vi "Initiate Measurement.vi"(0 "RS232 Port In":refnum<visa-resource-name>="COM1", 1 "Sensor Address In":string="0", 2 "Measurement Type In (Normal)":i32(ring) items=["Normal", "Concurrent", "Continuous"], 5 "Error In (No Error)":errorcluster, 6 "CRC In (False)":bool, 8 "Parameter In (0)":i32(ring) items=["0", "1", "2", "3", "4", "5", "6", "7", "8", "9"]) -> (10 "Parameter Out":i32(ring) items=["0", "1", "2", "3", "4", "5", "6", "7", "8", "9"], 12 "CRC Out":bool, 14 "RS232 Port Out":refnum<visa-resource-name>="COM1", 15 "Sensor Address Out":string="a", 16 "Measurement Type Out":i32(ring) items=["Normal", "Concurrent", "Continuous"], 17 "Number of Measurements":i32, 18 "Max Acquisition Time (sec)":i32, 19 "Error Out":errorcluster)   [LabVIEW 2016, in "SDI-12.lvlib"]
doc: "Creates and sends the Start Measurement command to the sensor. Scans the sensor's reply for the maximum amount of time for the measurement to complete, and the number of measurements that it will return.\n\nThis VI should only be called for Normal and Concurrent Measurements. Do not call with Continuous Measurements."
uses:
  SDI-12.lvlib
panel:
  out "loop":i32
  out "read buffer":string
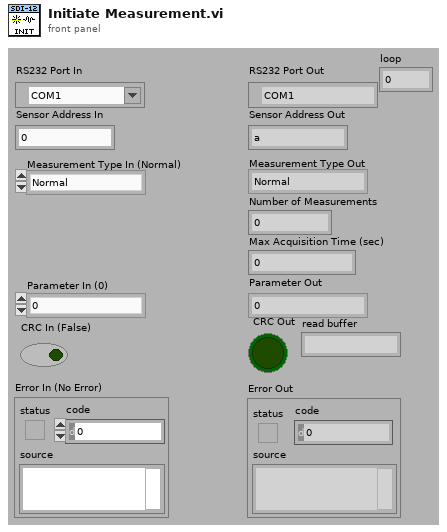
[diagram p1: front panel]
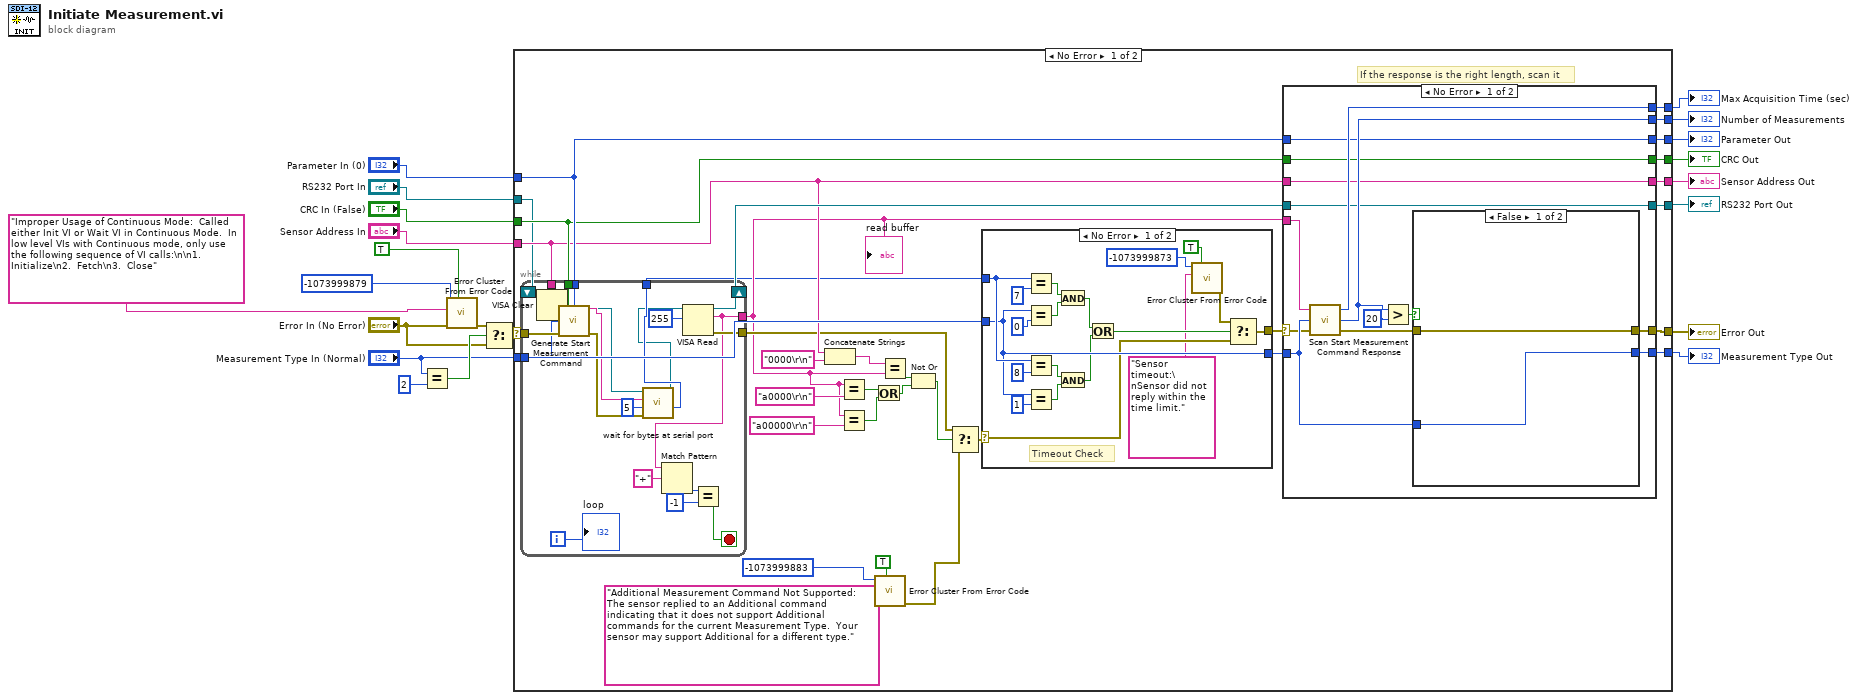
[diagram p0: block diagram]
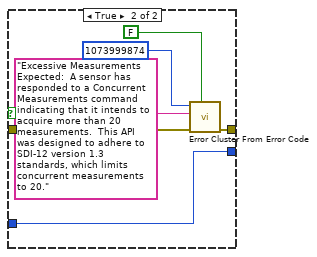
[diagram p3: hidden frame]
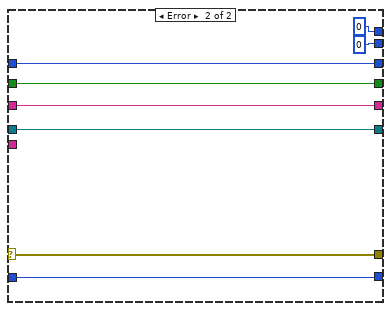
[diagram p4: hidden frame]
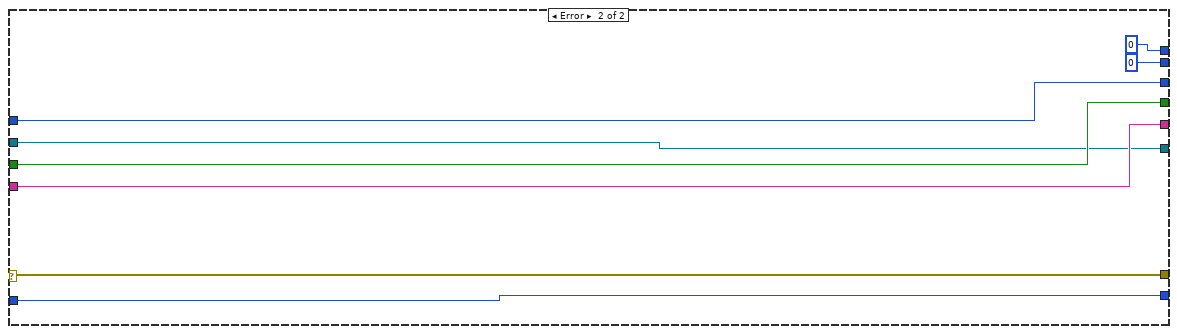
[diagram p5: hidden frame]
diagram:
  n1 = Equal?(x="Measurement Type In (Normal)", y=2) -> (x = y?=w16:bool)
  n2 = call <vilib>:"Error Cluster From Error Code.vi"("show call chain? (False)"=TRUE ("Error?"), "error in (no error)"="Error In (No Error)", "error message (\"\")"="Improper Usage of Continuous Mode:  Called either Init VI or Wait VI in Continuous Mode.  In low level VIs with Continuous mode, only use the following sequence of VI calls:\n\n1.  Initialize\n2.  Fetch\n3.  Close" ("error message (\"\")"), "error code (0)"=-1073999879 ("error code")) -> ("error out"=w15:errorcluster)  [unwired: 5 in]
  n3 = Select(t=w15, s=w16, f="Error In (No Error)") -> (s? t:f=w14:errorcluster)
  n4 = case shown="No Error" w14 {
    selector: w14 -> [w55 w135]
    tunnel: [w54 w135] -> w21
    tunnel: "Measurement Type In (Normal)" -> [w34 w134]
    tunnel: "RS232 Port In" -> [w22 w128]
    tunnel: "Parameter In (0)" -> [w50 w131]
    tunnel: "CRC In (False)" -> [w48 w130]
    tunnel: "Sensor Address In" -> [w31 w129]
    tunnel: [w53 w134] -> w7
    tunnel: [w52 0 ("Number of Measurements")] -> w6
    tunnel: [w51 0 ("Max Acquisition Time")] -> w5
    tunnel: [w49 w131] -> w4
    tunnel: [w47 w130] -> w3
    tunnel: [w46 w129] -> w2
    tunnel: [w44 w128] -> w1
    frame No Error {
      # "If the response is the right length, scan it"
      n5 = while {
        tunnel: w55 -> [w76]
        tunnel: w50 -> [w74]
        tunnel: w48 -> [w73]
        tunnel: w34 -> [w71]
        tunnel: w31 -> [w70]
        tunnel: [w69] -> w29
        tunnel: [w62] -> w28
        tunnel: [w68] -> w23
        shift-right: [w72] -> w45
        shift-left: w22 -> [w66]
        i -> [w57]
        stop <- w58 stop-if-true
        n6 = VISA Clear(VISA resource name=w66) -> (VISA resource name out=w56:refnum<visa-resource-name>)  [unwired: 1 in, 1 out]
        n7 = call "Generate Start Measurement Command.vi"("Sensor Address In"=w70, "CRC (False)"=w73, "Parameter (0)"=w74, "Measurement Type In (Normal)"=w71, "Error In (No Error)"=w76) -> ("Command"=w64:string, "Error Out"=w65:errorcluster)  [unwired: 9 in]
        n8 = call "wait for bytes at serial port.vi"("error in (no error)"=w65, "lower limit"=5, "String"=w64, "VISA Refnum in"=w56) -> ("return count"=w68:u32, "VISA Refnum out"=w67:refnum<visa-resource-name>)  [unwired: 4 in, 2 out]
        n9 = VISA Read(VISA resource name=w67, byte count=u32 255) -> (VISA resource name out=w72:refnum<visa-resource-name>, read buffer=w62:string, error out=w69:errorcluster)  [unwired: 1 in, 1 out]
        n10 = Match Pattern(string=w62, regular expression="+") -> (offset past match=w60:i32)  [unwired: 1 in, 3 out]
        n11 = Equal?(x=w60, y=-1) -> (x = y?=w58:bool)
        "loop" <- w57
      }
      "read buffer" <- w28
      n12 = Concatenate Strings(w31, "0000\r\n") -> (w38:string)
      n13 = Equal?(x=w28, y="a0000\r\n" ("read buffer")) -> (x = y?=w26:bool)
      n14 = Equal?(x=w28, y="a00000\r\n" ("read buffer")) -> (x = y?=w25:bool)
      n15 = Or(x=w26, y=w25) -> (x .or. y?=w24:bool)
      n16 = call <vilib>:"Error Cluster From Error Code.vi"("show call chain? (False)"=TRUE, "error message (\"\")"="Additional Measurement Command Not Supported:  The sensor replied to an Additional command indicating that it does not support Additional commands for the current Measurement Type.  Your sensor may support Additional for a different type." ("error message (\"\")"), "error code (0)"=-1073999883 ("error code")) -> ("error out"=w30:errorcluster)  [unwired: 6 in]
      n17 = Equal?(x=w38, y=w28) -> (x = y?=w37:bool)
      n18 = Not Or(1:w24, 2:w37) -> (0:w36:bool)
      n19 = Select(t=w29, s=w36, f=w30) -> (s? t:f=w35:errorcluster)
      n20 = case shown="No Error" w35 {
        selector: w35 -> [w83 w96]
        tunnel: w23 -> [w89 _]
        tunnel: w34 -> [w87 w97]
        tunnel: [w87 w97] -> w33
        tunnel: [w77 w96] -> w32
        frame No Error {
          # "Timeout Check"
          n21 = Equal?(x=w89, y=u32 7) -> (x = y?=w94:bool)
          n22 = Equal?(x=w87, y=0) -> (x = y?=w92:bool)
          n23 = Equal?(x=w89, y=u32 8) -> (x = y?=w91:bool)
          n24 = Equal?(x=w87, y=1) -> (x = y?=w90:bool)
          n25 = And(x=w94, y=w92) -> (x .and. y?=w85:bool)
          n26 = And(x=w91, y=w90) -> (x .and. y?=w84:bool)
          n27 = Or(x=w85, y=w84) -> (x .or. y?=w82:bool)
          n28 = call <vilib>:"Error Cluster From Error Code.vi"("show call chain? (False)"=TRUE ("Error?"), "error message (\"\")"="Sensor timeout:\nSensor did not reply within the time limit." ("error message (\"\")"), "error code (0)"=-1073999873 ("error code")) -> ("error out"=w78:errorcluster)  [unwired: 6 in]
          n29 = Select(t=w78, s=w82, f=w83) -> (s? t:f=w77:errorcluster)
        }
        frame Error {
        }
      }
      n30 = case shown="No Error" w32 {
        selector: w32 -> [w98 w120]
        tunnel: w28 -> [w109 _]
        tunnel: w33 -> [w106 w121]
        tunnel: [w107 w120] -> w54
        tunnel: [w105 w121] -> w53
        tunnel: [w104 0 ("Number of Measurements")] -> w52
        tunnel: [w103 0 ("Max Acquisition Time")] -> w51
        tunnel: w50 -> [w102 w125]
        tunnel: [w102 w125] -> w49
        tunnel: w48 -> [w101 w124]
        tunnel: [w101 w124] -> w47
        tunnel: w31 -> [w100 w122]
        tunnel: [w100 w122] -> w46
        tunnel: w45 -> [w99 w123]
        tunnel: [w99 w123] -> w44
        frame No Error {
          n31 = call "Scan Start Measurement Command Response.vi"("Error In (No Error)"=w98, "Measurement Type In (Normal)"=w106, "Measurement Response"=w109) -> ("Error Out"=w108:errorcluster, "Number of Measurements"=w104:i32, "Max Acquisition Time"=w103:i32)
          n32 = Greater?(x=w104, y=20) -> (0:w110:bool)
          n33 = case shown="False" w110 {
            tunnel: [w113 w116] -> w107
            tunnel: w108 -> [w113 w115]
            tunnel: w106 -> [w112 w114]
            tunnel: [w112 w114] -> w105
            frame False {
            }
            frame True {
              n34 = call <vilib>:"Error Cluster From Error Code.vi"("show call chain? (False)"=FALSE ("Error?"), "error in (no error)"=w115, "error message (\"\")"="Excessive Measurements Expected:  A sensor has responded to a Concurrent Measurements command indicating that it intends to acquire more than 20 measurements.  This API was designed to adhere to SDI-12 version 1.3 standards, which limits concurrent measurements to 20." ("error message (\"\")"), "error code (0)"=1073999874 ("error code")) -> ("error out"=w116:errorcluster)  [unwired: 5 in]
            }
          }
        }
        frame Error {
        }
      }
    }
    frame Error {
    }
  }
  "Error Out" <- w21
  "Measurement Type Out" <- w7
  "Number of Measurements" <- w6
  "Max Acquisition Time (sec)" <- w5
  "Parameter Out" <- w4
  "CRC Out" <- w3
  "Sensor Address Out" <- w2
  "RS232 Port Out" <- w1
